vi "Configure Ltest Measurement.vi"(4 "Enables Limit Test (T: Enable)":bool=TRUE, 5 "Percent Margin (0)":dbl, 6 "Fail Condition (0: Inside)":i32(ring) items=["Inside", "Outside"], 7 "Upper Limit (0)":dbl, 8 "error in (no error)":errorcluster, 9 "Lower Limit (0)":dbl, 10 "Measurement Source (MEAS1)":i32(ring) items=["MEAS1", "MEAS2", "MEAS3", "MEAS4", "MEAS5", "MEAS6", "MEAS7", "MEAS8", "MEAS9", "MEAS10"], 11 "VISA resource name":refnum<visa-resource-name>) -> (0 "error out":errorcluster, 3 "VISA resource name out":refnum<visa-resource-name>)   [LabVIEW 2015, in "Agilent 2000 3000 X-Series.lvlib"]
doc: "Configures the ltest measurement"
uses:
  Agilent 2000 3000 X-Series.lvlib
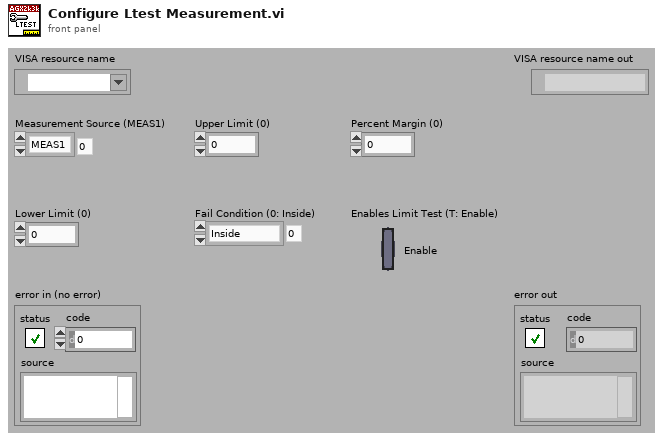
[diagram p1: front panel]
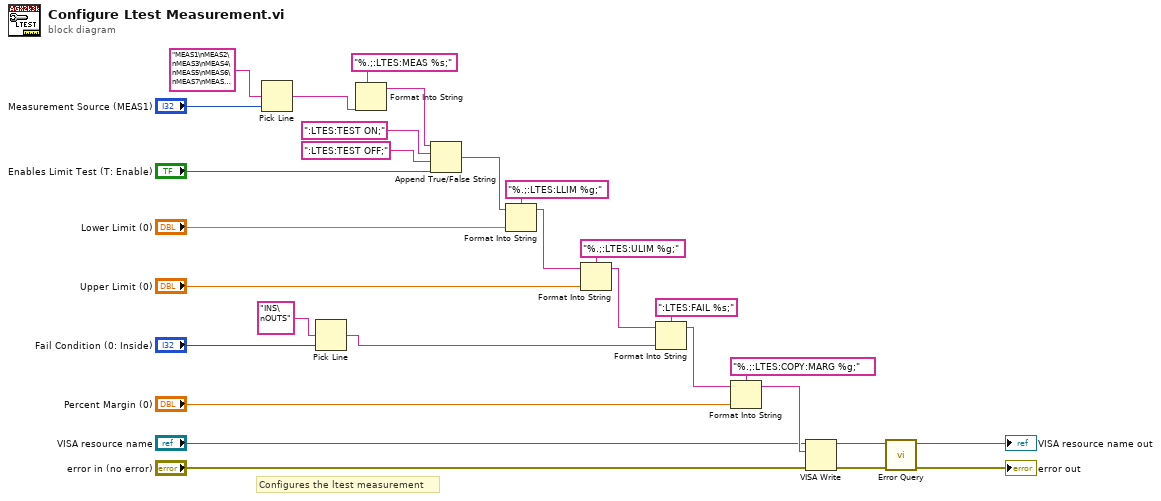
[diagram p0: block diagram]
diagram:
  # "Configures the ltest measurement"
  n1 = Pick Line(multi-line string="MEAS1\nMEAS2\nMEAS3\nMEAS4\nMEAS5\nMEAS6\nMEAS7\nMEAS8\nMEAS9\nMEAS10", line index="Measurement Source (MEAS1)") -> (output string=w2:string)  [unwired: 1 in]
  n2 = Pick Line(multi-line string="INS\nOUTS", line index="Fail Condition (0: Inside)") -> (output string=w4:string)  [unwired: 1 in]
  n3 = Format Into String(format string="%.;:LTES:MEAS %s;", w2) -> (resulting string=w28:string)  [unwired: 2 in, 1 out]
  n4 = Append True/False String(1:"Enables Limit Test (T: Enable)", 2:":LTES:TEST OFF;", 3:":LTES:TEST ON;", 4:w28) -> (0:w24:string)
  n5 = Format Into String(format string="%.;:LTES:LLIM %g;", initial string=w24, "Lower Limit (0)") -> (resulting string=w21:string)  [unwired: 1 in, 1 out]
  n6 = Format Into String(format string="%.;:LTES:ULIM %g;", initial string=w21, "Upper Limit (0)") -> (resulting string=w18:string)  [unwired: 1 in, 1 out]
  n7 = Format Into String(format string=":LTES:FAIL %s;", initial string=w18, w4) -> (resulting string=w16:string)  [unwired: 1 in, 1 out]
  n8 = Format Into String(format string="%.;:LTES:COPY:MARG %g;", initial string=w16, "Percent Margin (0)") -> (resulting string=w13:string)  [unwired: 1 in, 1 out]
  n9 = VISA Write(VISA resource name="VISA resource name", write buffer=w13, error in (no error)="error in (no error)") -> (VISA resource name out=w10:refnum<visa-resource-name>, error out=w7:errorcluster)  [unwired: 1 out]
  n10 = call "Error Query.vi"("error in (no error)"=w7, "VISA resource name"=w10) -> ("error out"=→"error out":errorcluster, "VISA resource name out"=→"VISA resource name out":refnum<visa-resource-name>)  [unwired: 6 in, 2 out]
